vi "CgtpWriteVariableAsInteger.vi"(0 "error in":errorcluster, 1 "progName":string, 5 "Cgtp":refnum<k24>, 7 "varName":string, 9 "value":i32) -> (4 "error out":errorcluster)   [LabVIEW 2022 SP3, in "UnderAutomation.Fanuc.lvlib"]
uses:
  UnderAutomation.Fanuc.lvlib
  C:/Users/fg/Documents/Fanuc.vi/LabVIEW_2024/UnderAutomation.Fanuc/lib/UnderAutomation.Fanuc.dll
  LabVIEW_2024/UnderAutomation.Fanuc/lib/UnderAutomation.Fanuc.dll
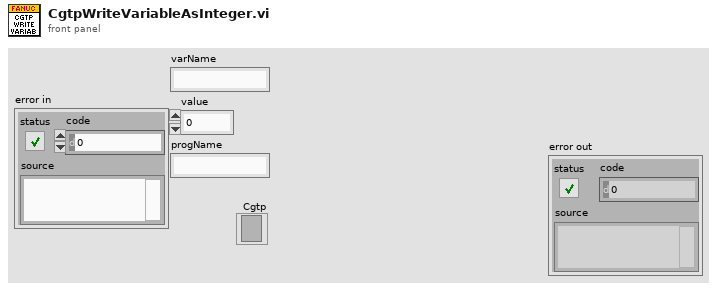
[diagram p1: front panel]
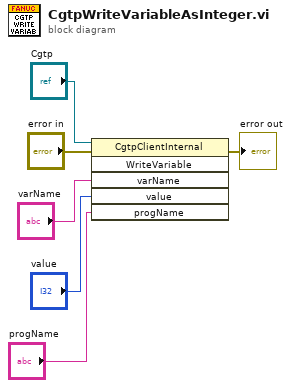
[diagram p0: block diagram]
diagram:
  n1 = invoke class="CgtpClientInternal" method="WriteVariable"(reference="Cgtp", error in="error in", "varName"="varName", "value"="value", "progName"="progName") -> (error out=→"error out":errorcluster)  [unwired: 1 in, 5 out]
